vi "rotate_2D_array.vi"(7 "transpose?":bool, 10 "array":dbl[][](array[numeric]), 11 "n":i32) -> (2 "array_rotated":dbl[][](array[numeric]))   [LabVIEW 2015, in "lv-graph-global.lvlib"]
uses:
  lv-graph-global.lvlib
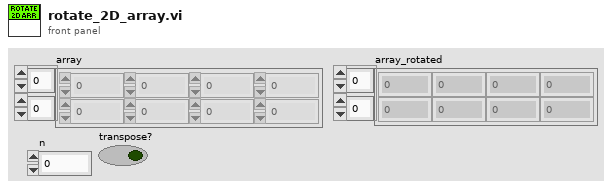
[diagram p1: front panel]
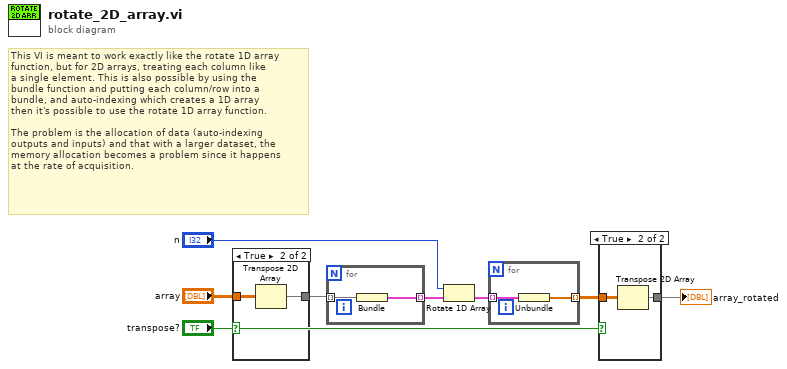
[diagram p0: block diagram]
diagram:
  # "This VI is meant to work exactly like the rotate 1D array\nfunction, but for 2D arrays, treating each column like\na single element. This is also possible by using the\nbundle function and putting each column/row into a\nbundle, and auto-indexing which creates a 1D array\nthen it's possible to use the rotate 1D array function.\n\nThe problem is the allocation of data (auto-indexing\noutputs and inputs) and that with a larger dataset, the\nmemory allocation becomes a problem since it happens\nat the rate of acquisition."
  n1 = case shown="True" "transpose?" {
    tunnel: "array" -> [w9 w11]
    tunnel: [w9 w10] -> w1
    frame False {
    }
    frame True {
      n2 = Transpose 2D Array(2D array=w11) -> (transposed array=w10:dbl[][])
    }
  }
  n3 = for {
    tunnel: w1 -> [w13] mode=indexing
    tunnel: [w12] -> w3 mode=indexing
    n4 = Bundle("array"=w13) -> (w12:cluster{"array":dbl[]})  [unwired: 1 in]
  }
  n5 = Rotate 1D Array(1:w3, 2:"n") -> (0:w4:cluster{"array":dbl[]}[])
  n6 = for {
    tunnel: w4 -> [w15] mode=indexing
    tunnel: [w14] -> w2 mode=indexing
    n7 = Unbundle(w15) -> ("array"=w14:dbl[])
  }
  n8 = case shown="True" "transpose?" {
    tunnel: w2 -> [w16 w18]
    tunnel: [w16 w17] -> w6
    frame False {
    }
    frame True {
      n9 = Transpose 2D Array(2D array=w18) -> (transposed array=w17:dbl[][])
    }
  }
  "array_rotated" <- w6
